vi "Create Value - Boolean.vi"(8 "error in (no error)":errorcluster, 10 "Boolean":bool) -> (0 "error out":errorcluster, 3 "JSON Tree":variant)   [LabVIEW 2013, in "i3-json.lvlib"]
doc: "Creates a new JSON Object of the given type"
uses:
  i3-json.lvlib
  JSON Types/JSON Type.ctl
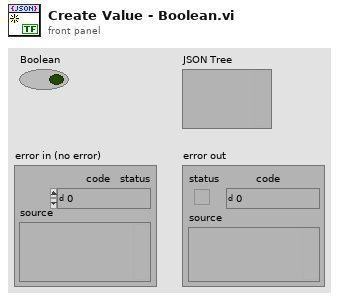
[diagram p1: front panel]
types:
  T1 = typedef "i3-json.lvlib/JSON Type.ctl" = enum8{"JSON Compatible", "JSON Array", "JSON Object", "JSON Null", "Double", "String", "Boolean", "Unknown"}
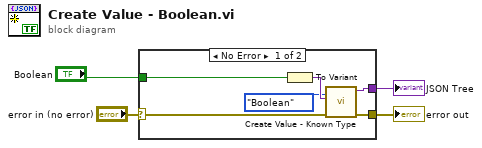
[diagram p0: block diagram]
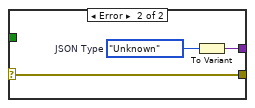
[diagram p2: hidden frame]
diagram:
  n1 = case shown="No Error" "error in (no error)" {
    selector: "error in (no error)" -> [w8 w11]
    tunnel: [w9 w11] -> w3
    tunnel: [w10 w12] -> w2
    tunnel: "Boolean" -> [w5 _]
    frame No Error {
      n2 = To Variant(anything=w5) -> (Variant=w7:variant)
      n3 = call "Create Value - Known Type.vi"("JSON Type"=JSON_Type."Boolean", "error in (no error)"=w8, "Value"=w7) -> ("error out"=w9:errorcluster, "JSON Tree"=w10:variant)  [unwired: 7 in]
    }
    frame Error {
      w13 = JSON_Type."Unknown"  # JSON Type
      n4 = To Variant(anything=w13) -> (Variant=w12:variant)
    }
  }
  "JSON Tree" <- w2
  "error out" <- w3
